vi "Initialize Bus Settings.vi"(8 "error in (no error)":errorcluster, 9 "XNET Settings":T1={"Port"="", "Baud Rate"=0, "Termination"=0, "CAN I/O Mode"=0, "FD Baud Rate"=500000, "Priority"=100, "FD ISO Mode"=0} {"FD ISO Mode" items=["ISO", "Non ISO", "ISO Legacy"]; "CAN I/O Mode" items=["CAN 2.0", "CAN FD", "CAN FD+BRS"]; "Termination" items=["Off", "On"]}, 10 "XNET Refs":T2, 11 "Bus Info":T4) -> (0 "error out":errorcluster, 3 "Bus Settings":T3={"Name"="", "Overrides?"=FALSE, "XNET Refs"={"Incoming"="", "Outgoing"=""}, "Port Info"={"Port"="", "Baud Rate"=0, "Termination"=0, "CAN I/O Mode"=0, "FD Baud Rate"=500000, "Priority"=100, "FD ISO Mode"=0}, "Frames"=variant(cluster{"Convert Session":refnum<k21>, "ID":u32, "Length":i32, "Offset":i32}[] [])} {"Port Info"."FD ISO Mode" items=["ISO", "Non ISO", "ISO Legacy"]; "Port Info"."CAN I/O Mode" items=["CAN 2.0", "CAN FD", "CAN FD+BRS"]; "Port Info"."Termination" items=["Off", "On"]})   [LabVIEW 2019, in "Ghost Bus Addon Engine.lvlib"]
uses:
  Ghost Bus Addon Engine.lvlib
  Addon Shared/Types/Exported.Bus.Settings.ctl
  Addon Shared/Types/Exported.Frames.Settings.ctl
  Addon Shared/Types/Frame Settings.ctl
  Types/RT Bus Settings.ctl
  Types/RT XNET Refs.ctl
  Addon Shared/Types/XNET Port Settings.ctl
  Types/RT Frame Settings.ctl
  <vilib>/xnet/xnet.llb/XNET Create Session (Conversion).vi
  Addon Shared/Ghost Bus Addon Shared.lvlib
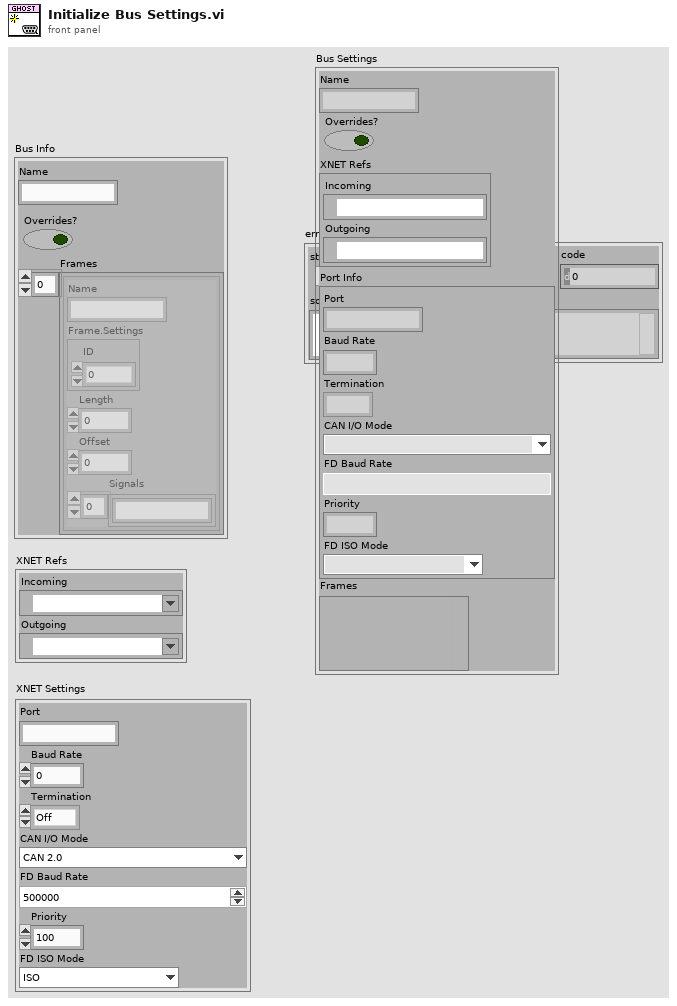
[diagram p1: front panel]
types:
  T1 = typedef "Ghost Bus Addon Shared.lvlib/XNET Port Settings.ctl" = cluster{"Port":string, "Baud Rate":u64, "Termination":u32, "CAN I/O Mode":u32, "FD Baud Rate":u64, "Priority":i32, "FD ISO Mode":u32}
  T2 = typedef "Ghost Bus Addon Engine.lvlib/RT XNET Refs.ctl" = cluster{"Incoming":refnum<k21>, "Outgoing":refnum<k21>}
  T3 = typedef "RT Bus Settings.ctl" = cluster{"Name":string, "Overrides?":bool, "XNET Refs":T2, "Port Info":T1, "Frames":variant}
  T4 = typedef "Ghost Bus Addon Shared.lvlib/Exported.Bus.Settings.ctl" = cluster{"Name":string, "Overrides?":bool, "Frames":T5[]}
  T5 = typedef "Ghost Bus Addon Shared.lvlib/Exported.Frames.Settings.ctl" = cluster{"Name":string, "Frame.Settings":T6, "Length":i32, "Offset":i32, "Signals":string[]}
  T6 = typedef "Ghost Bus Addon Shared.lvlib/Frame Settings.ctl" = cluster{"ID":u32}
  T7 = typedef "Ghost Bus Addon Engine.lvlib/RT Frame Settings.ctl" = cluster{"Convert Session":refnum<k21>, "Length":i32, "Offset":i32, "Enable Offset":i32}
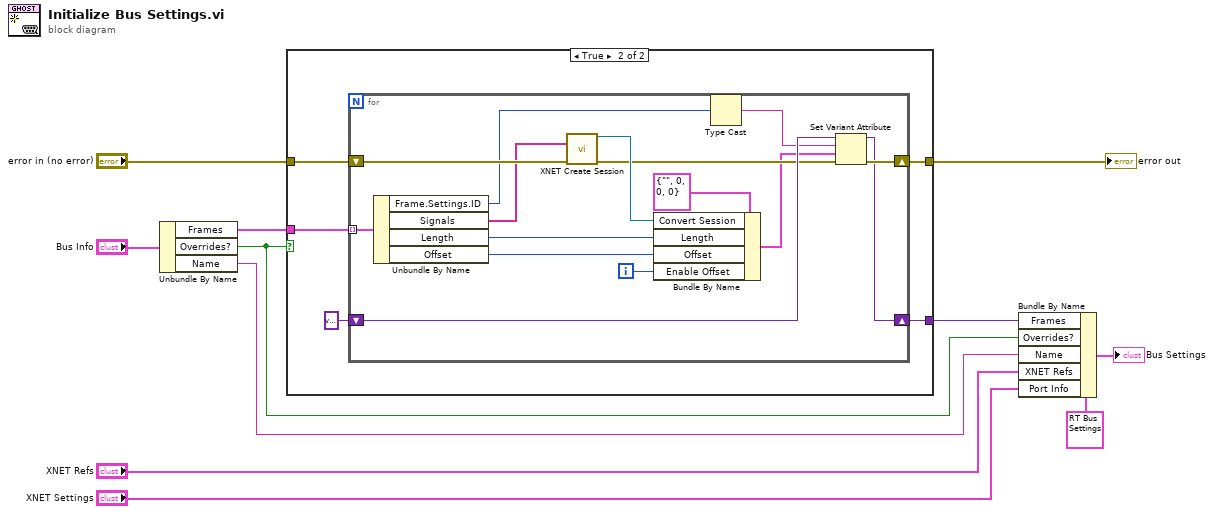
[diagram p0: block diagram]
diagram:
  n1 = Unbundle By Name("Bus Info") -> ("Frames"=w10:T5[], "Overrides?"=w7:bool, "Name"=w6:string)
  n2 = case shown="True" w7 {
    tunnel: "error in (no error)" -> [w12 w17]
    tunnel: w10 -> [_ w16]
    tunnel: [w12 w15] -> w9
    tunnel: [_ w13] -> w8
    frame False {
    }
    frame True {
      n3 = for {
        shift-right: [w23] -> w15
        shift-left: w17 -> [w32]
        tunnel: w16 -> [w31] mode=indexing
        shift-right: [w22] -> w13
        shift-left: variant -> [w25]
        i -> [w18]
        n4 = Unbundle By Name(w31) -> ("Frame.Settings.ID"=w19:u32, "Signals"=w30:string[], "Length"=w28:i32, "Offset"=w27:i32)
        n5 = call-poly <vilib>:"XNET Create Session.vi"("signal list"=w30, "error in (no error)"=w32) -> ("session out"=w29:refnum<k21>, "error out"=w24:errorcluster)  [unwired: 12 in]
        n6 = Bundle By Name(cluster=T7 {"Convert Session"="", "Length"=0, "Offset"=0, "Enable Offset"=0}, "Convert Session"=w29, "Length"=w28, "Offset"=w27, "Enable Offset"=w18) -> (w21:T7)
        n7 = Type Cast(x=w19) -> (*(type *) &x=w20:string)  [unwired: 1 in]
        n8 = Set Variant Attribute(Variant=w25, name=w20, value=w21, error in=w24) -> (Variant out=w22:variant, error out=w23:errorcluster)  [unwired: 1 out]
      }
    }
  }
  "error out" <- w9
  n9 = Bundle By Name(cluster=T3 {"Name"="", "Overrides?"=FALSE, "XNET Refs"={"Incoming"="", "Outgoing"=""}, "Port Info"={"Port"="", "Baud Rate"=0, "Termination"=0, "CAN I/O Mode"=0, "FD Baud Rate"=500000, "Priority"=100, "FD ISO Mode"=0}, "Frames"=variant(cluster{"Convert Session":refnum<k21>, "ID":u32, "Length":i32, "Offset":i32}[] [])}, "Frames"=w8, "Overrides?"=w7, "Name"=w6, "XNET Refs"="XNET Refs", "Port Info"="XNET Settings") -> (→"Bus Settings":T3)
